vi "ex4.vi"() -> ()   [LabVIEW 2020]
uses:
  <vilib>/measure/madcrms.llb/Basic Averaged DC-RMS for N Chan.vi
  <vilib>/measure/NI_MAPro.lvlib
panel:
  out "amlitude":dbl
  out "frequency":dbl
  out "ofset":dbl
  out "Waveform Graph":dynamicdata(graph)
  in  "samples":dbl
  in  "Fs":dbl
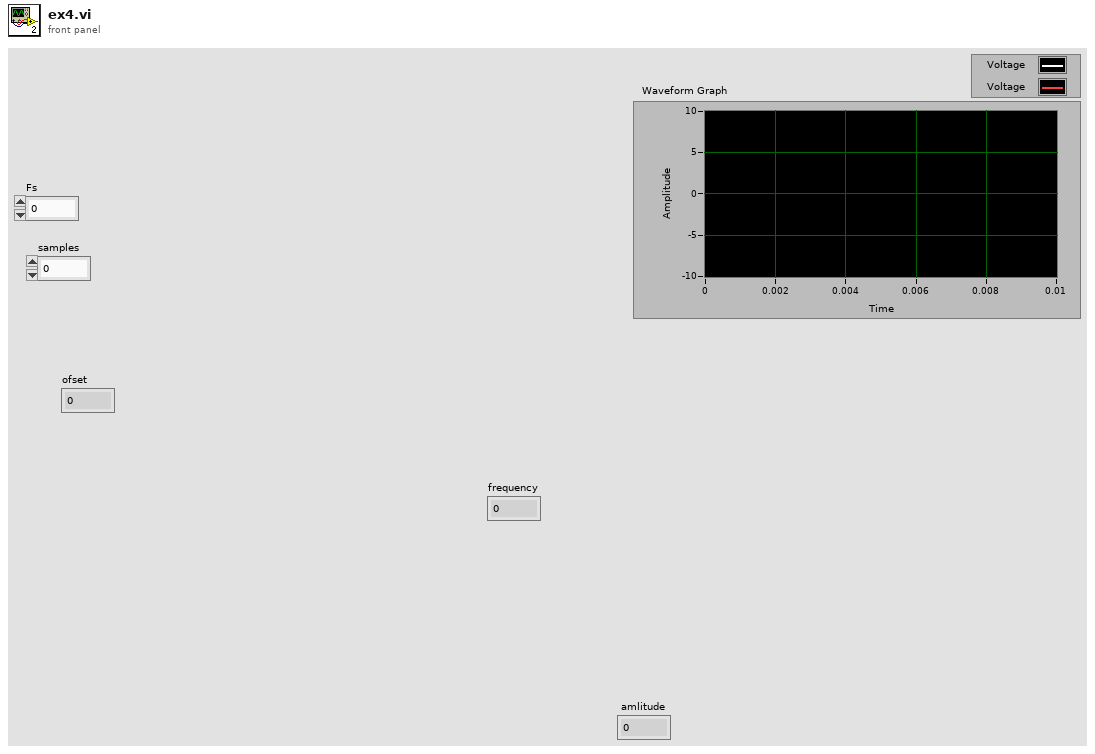
[diagram p1: front panel]
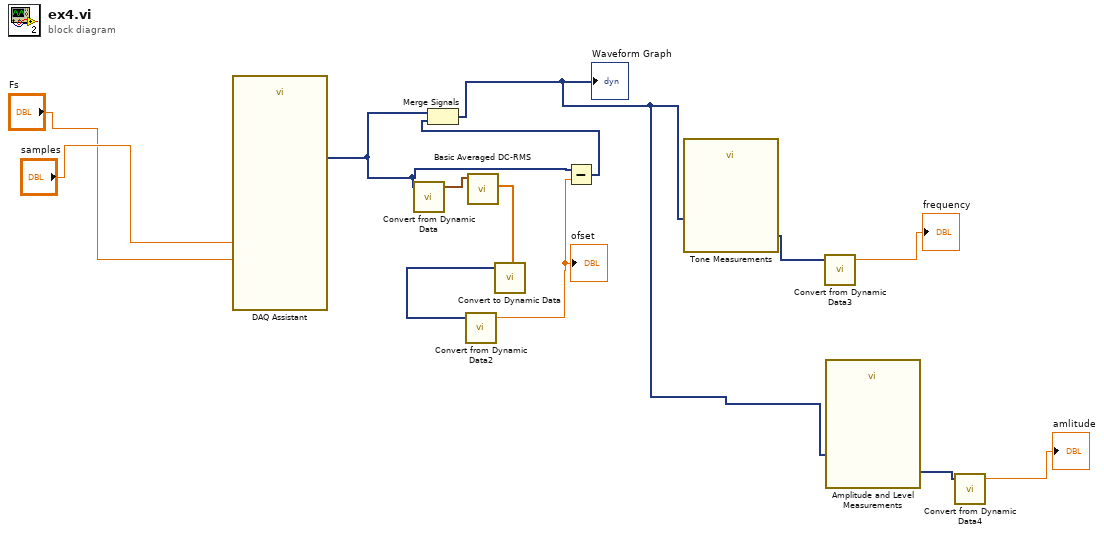
[diagram p0: block diagram]
diagram:
  n1 = call "DAQ Assistant"("rate"="Fs", "number of samples"="samples") -> ("data"=w12:dynamicdata)  [unwired: 15 in, 2 out]
  n2 = call "Convert from Dynamic Data"("Dynamic Data Type"=w12) -> ("Array of Waveform"=w11:waveform(dbl)[])  [unwired: 3 in]
  n3 = call-poly <vilib>:"Basic Averaged DC-RMS.vi"("signals in"=w11) -> ("RMS values"=w10:dbl[])  [unwired: 7 in, 3 out]
  n4 = call "Convert to Dynamic Data"("Array"=w10) -> ("Dynamic Data Type"=w9:dynamicdata)  [unwired: 3 in]
  n5 = call "Convert from Dynamic Data2"("Dynamic Data Type"=w9) -> ("Scalar"=w8:dbl)  [unwired: 3 in]
  "ofset" <- w8
  n6 = Subtract(x=w12, y=w8) -> (x-y=w7:dynamicdata)
  n7 = Merge Signals(w12, w7) -> (w6:dynamicdata)
  "Waveform Graph" <- w6
  n8 = call "Tone Measurements"("Signals"=w6) -> ("Frequency"=w5:dynamicdata)  [unwired: 9 in, 1 out]
  n9 = call "Convert from Dynamic Data3"("Dynamic Data Type"=w5) -> ("Scalar"=→"frequency":dbl)  [unwired: 3 in]
  n10 = call "Amplitude and Level Measurements"("Signals"=w6) -> ("Peak to Peak"=w2:dynamicdata)  [unwired: 13 in, 1 out]
  n11 = call "Convert from Dynamic Data4"("Dynamic Data Type"=w2) -> ("Scalar"=→"amlitude":dbl)  [unwired: 3 in]
